vi "Scope Trace Get Trigger Level.vi"(11 "Waveform Data":waveform(dbl)={"t0"=timestamp(-0.5 s since 1904-01-01), "dt"=0.0004, "Y"=array[2500 elements]}) -> (1 "Waveform Graph 2":waveform(dbl)(graph), 2 "XY Graph":cluster{"X":dbl[], "Y":dbl[]}[](graph), 3 "max value":dbl)   [LabVIEW 2020]
uses:
  <vilib>/Analysis/1siggen.llb/Ramp Pattern by Samples.vi
  <vilib>/measure/mamon.llb/Waveform Peak Detection for 1 Chan.vi
  <vilib>/measure/NI_MAPro.lvlib
  <vilib>/Analysis/NI_AAL_SigProc.lvlib
  <vilib>/Analysis/NI_AALBase.lvlib
panel:
  in  "Y":dbl[](array[numeric])
  out "Peak to Peak":dbl
  out "Positive Peak":dbl
  out "max":dbl format="%.4f"
  out "Waveform Graph 3":dbl[](graph)
  out "RMS":dbl format="%0.2f"
  out "Waveform Graph":dbl[](graph)
  out "Amplitudes":dbl[](array[numeric]) format="%.2p"
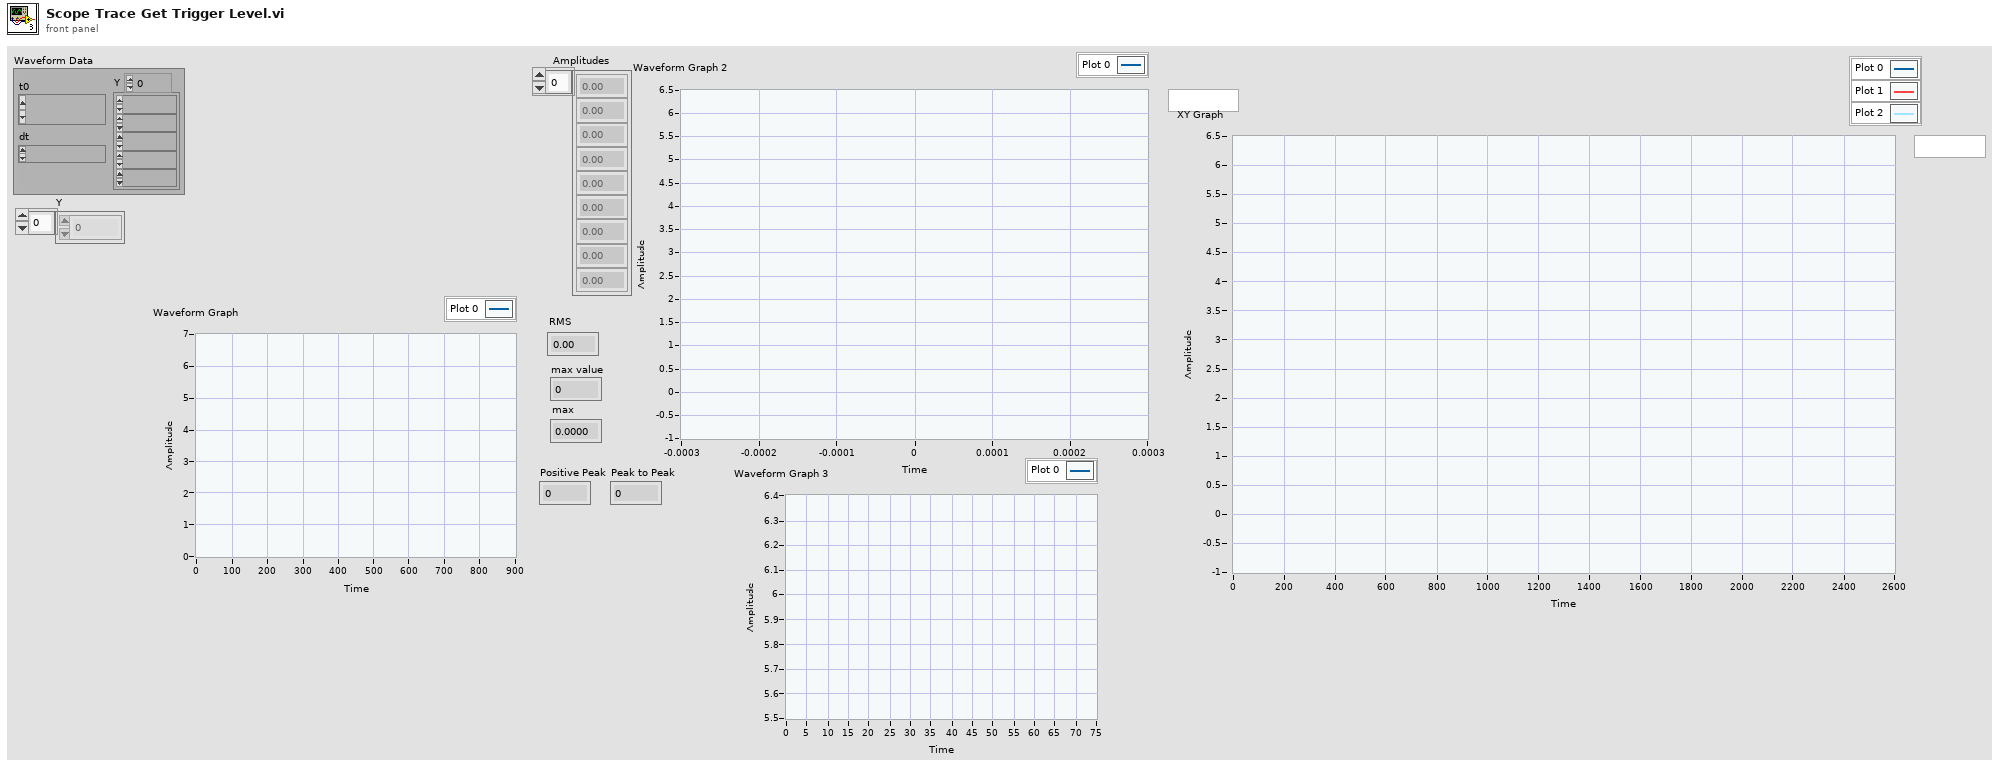
[diagram p1: front panel]
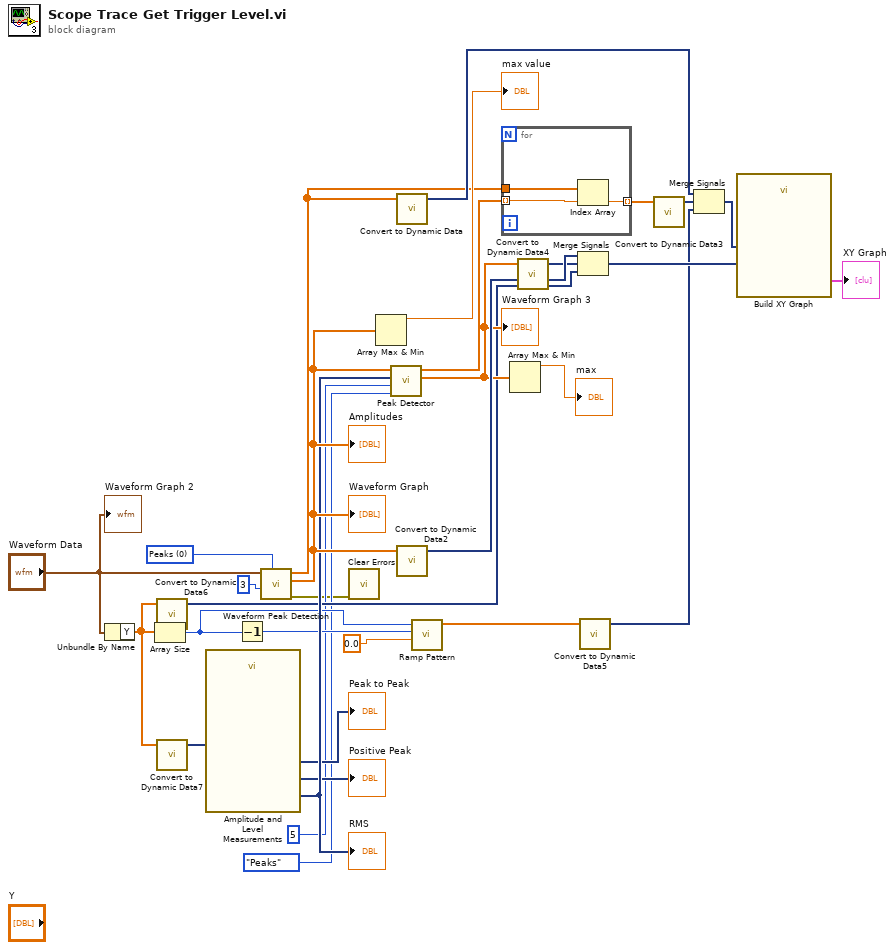
[diagram p0: block diagram]
diagram:
  w31 = u16 0 items=["Peaks", "Valleys"] ("peaks/valleys")
  n1 = Unbundle By Name("Waveform Data") -> ("Y"=w3:dbl[])
  n2 = Array Size(array=w3) -> (size(s)=w12:i32)
  n3 = call "Convert to Dynamic Data6"("Array"=w3) -> ("Dynamic Data Type"=w8:dynamicdata)  [unwired: 3 in]
  n4 = call "Convert to Dynamic Data7"("Array"=w3) -> ("Dynamic Data Type"=w2:dynamicdata)  [unwired: 3 in]
  n5 = call "Amplitude and Level Measurements"("Signals"=w2) -> ("RMS"=w16:dynamicdata, "Positive Peak"=→"Positive Peak":dynamicdata, "Peak to Peak"=→"Peak to Peak":dynamicdata)  [unwired: 11 in, 1 out]
  "RMS" <- w16
  n6 = Decrement(x=w12) -> (x-1=w11:i32)
  n7 = call-poly <vilib>:"Waveform Peak Detection.vi"("peaks/valleys"=w31, "width"=3, "Signal In"="Waveform Data") -> ("error out"=w1:errorcluster, "Amplitudes"=w27:dbl[], "Locations"=w18:dbl[])  [unwired: 4 in, 2 out]
  "Amplitudes" <- w27
  "Waveform Graph" <- w27
  n8 = call <vilib>:"Clear Errors.vi"("error in (no error)"=w1) -> ()  [unwired: 5 in, 2 out]
  n9 = Array Max & Min(array=w27) -> (max value=→"max value":dbl)  [unwired: 3 out]
  n10 = call <vilib>:"Peak Detector.vi"("peaks/valleys"=enum32{"Peaks", "Valleys"}."Peaks", "width"=5, "threshold"=w16, "X"=w27) -> ("Amplitudes"=w22:dbl[], "Locations"=w19:dbl[])  [unwired: 3 in, 3 out]
  "Waveform Graph 3" <- w22
  n11 = call "Convert to Dynamic Data"("Array"=w18) -> ("Dynamic Data Type"=w28:dynamicdata)  [unwired: 3 in]
  n12 = call "Convert to Dynamic Data2"("Array"=w27) -> ("Dynamic Data Type"=w26:dynamicdata)  [unwired: 3 in]
  n13 = call-poly <vilib>:"Ramp Pattern.vi"("start"=0.0, "end"=w11, "samples"=w12) -> ("Ramp Pattern"=w10:dbl[])  [unwired: 7 in, 1 out]
  n14 = for {
    tunnel: w19 -> [w33] mode=indexing
    tunnel: w18 -> [w34]
    tunnel: [w32] -> w17 mode=indexing
    n15 = Index Array(array=w34, index=w33) -> (element=w32:dbl)
  }
  n16 = Array Max & Min(array=w22) -> (max value=→"max":dbl)  [unwired: 3 out]
  n17 = call "Convert to Dynamic Data4"("Array"=w22) -> ("Dynamic Data Type"=w21:dynamicdata)  [unwired: 3 in]
  n18 = Merge Signals(w26, w21, w8) -> (w23:dynamicdata)
  n19 = call "Convert to Dynamic Data5"("Array"=w10) -> ("Dynamic Data Type"=w9:dynamicdata)  [unwired: 3 in]
  n20 = call "Convert to Dynamic Data3"("Array"=w17) -> ("Dynamic Data Type"=w24:dynamicdata)  [unwired: 3 in]
  n21 = Merge Signals(w28, w24, w9) -> (w25:dynamicdata)
  n22 = call "Build XY Graph"("Y Input"=w23, "X Input"=w25) -> ("XY Graph"=→"XY Graph":cluster{"X":dbl[], "Y":dbl[]}[])  [unwired: 8 in, 1 out]
  "Waveform Graph 2" <- "Waveform Data"
